vi "Actor Core.vi"(8 "error in":errorcluster, 11 "ThresholdProcess2D in":refnum<class "ThresholdProcessor2D.lvclass">) -> (0 "error out":errorcluster, 3 "Actor out":refnum<class "Actor.lvclass">)   [LabVIEW 2014, in "ThresholdProcessor2D.lvclass"]
doc: "(<B>Filename</B>: Actor Framework.lvlib:Actor.lvclass:Actor Core.vi)\n\nReceives messages to the actor, reacts to them, and initiates any error handling that may shut the actor down.\n\nDescendant classes may override this VI to append parallel tasks for the actor to complete while it handles messages. Overrides use the Call Parent Method node."
uses:
  ThresholdProcessor2D.lvclass
  Framework/Interfaces/Viewable Actor/Viewable Actor.lvclass
  <vilib>/ActorFramework/Actor/Actor.lvclass
  Framework/Interfaces/Observable Actor/Observable Actor.lvclass
  ThresholdProcessor2D Messages/Write Threshold2D Msg/Write Threshold2D Msg.lvclass
  Framework/Processor/AbstractProcessor2D/AbstractProcessor2D.lvclass
  Framework/Model/Data/Data2D/Data2D.lvclass
  Framework/Processor/AbstractProcessor2D/Data2D Cluster.ctl
panel:
  out "Data2D out":dbl[][](graph)
  out "Data2D in":dbl[][](graph)
  out "Stop":bool=TRUE
  in  "Threshold":dbl
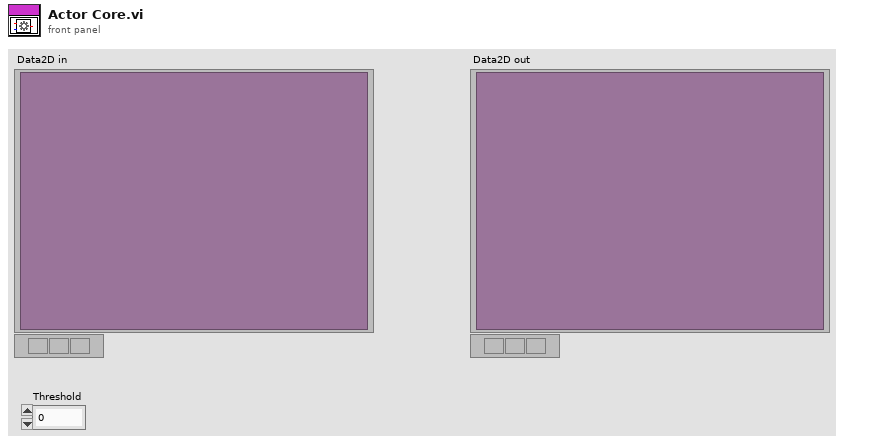
[diagram p1: front panel]
types:
  T1 = typedef "Observable Actor.lvlib/Observable Actor.lvclass/Observer.ctl" = refnum<queue>
  T2 = typedef "AbstractProcessor2D.lvclass/Data2D Cluster.ctl" = cluster{"in":refnum<class "Data2D.lvclass">, "out":refnum<class "Data2D.lvclass">}
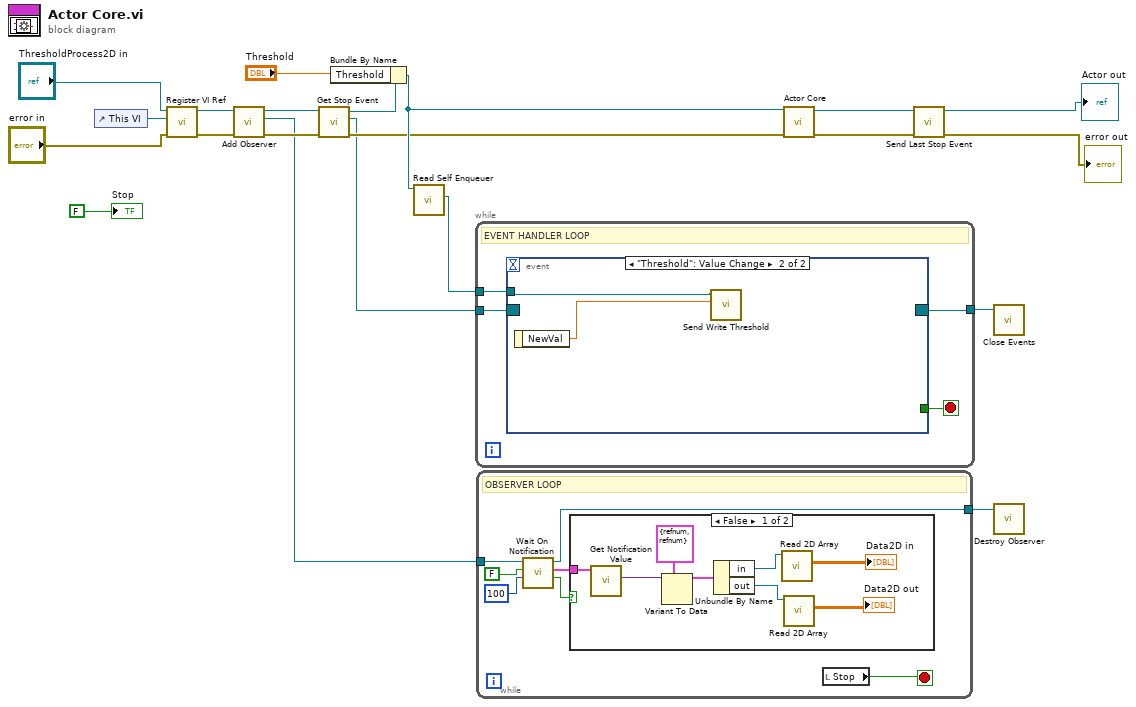
[diagram p0: block diagram]
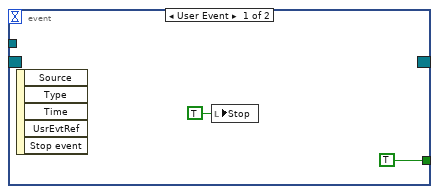
[diagram p3: hidden frame]
diagram:
  n1 = control-ref of="This VI"() -> (w21:refnum<vi>)
  n2 = call "Register VI Ref.vi"("error in (no error)"="error in", "VI ref"=w21, "Viewable Actor in"="ThresholdProcess2D in") -> ("error out"=w5:errorcluster, "Viewable Actor out"=w6:refnum<class "ThresholdProcessor2D.lvclass">)  [unwired: 7 in]
  n3 = call-dynamic "Add Observer.vi"("error in (no error)"=w5, "Observable Actor in"=w6) -> ("error out"=w4:errorcluster, "new observer"=w3:T1, "Observable Actor out"=w7:refnum<class "ThresholdProcessor2D.lvclass">)  [unwired: 7 in]
  n4 = call-dynamic "Get Stop Event.vi"("error in (no error)"=w4, "Observable Actor in"=w7) -> ("error out"=w9:errorcluster, "Events"=w8:refnum<event-registration>, "Observable Actor out"=w10:refnum<class "ThresholdProcessor2D.lvclass">)  [unwired: 7 in]
  n5 = Bundle By Name(cluster=w10, "Threshold"="Threshold") -> (w11:refnum<class "ThresholdProcessor2D.lvclass">)
  n6 = call <vilib>:"Read Self Enqueuer.vi"("Actor"=w11) -> ("Self Enqueuer"=w20:refnum<class "Message Enqueuer.lvclass">)  [unwired: 10 in]
  n7 = while {
    tunnel: w8 -> [w25]
    tunnel: w20 -> [w24]
    tunnel: [w23] -> w2
    stop <- w22 stop-if-true
    # "EVENT HANDLER LOOP"
    n8 = event shown="[1] \"Threshold\": Value Change" {
      selector: w25 -> [_ _]
      dyn-events: [_ _] -> w23
      timeout: _ -> [_ _]
      tunnel: w24 -> [_ w29]
      tunnel: [TRUE _] -> w22
      event User Event {
        n9 = event-data() -> ()  [unwired: 1 in, 5 out]
        n10 = local write "Stop"(TRUE ("Stop")) -> ()
      }
      event "Threshold": Value Change {
        n11 = event-data() -> ("NewVal"=w28:dbl)  [unwired: 1 in]
        n12 = call "Send Write Threshold.vi"("Threshold"=w28, "Message Enqueuer"=w29) -> ()  [unwired: 8 in, 2 out]
      }
    }
  }
  n13 = while {
    tunnel: [w34] -> w1
    tunnel: w3 -> [w35]
    stop <- w36 stop-if-true
    # "OBSERVER LOOP"
    n14 = call "Wait On Notification.vi"("timeout in ms (-1)"=100, "ignore previous (F)"=FALSE, "observer in"=w35) -> ("timed out?"=w30:bool, "notification"=w31:cluster{"value":variant, "name":string}, "observer out"=w34:T1)  [unwired: 5 in, 1 out]
    n15 = case shown="False" w30 {
      tunnel: w31 -> [w44 _]
      frame False {
        n16 = call "Get Notification Value.vi"("notification in"=w44) -> ("data"=w41:variant)  [unwired: 7 in, 1 out]
        n17 = Variant To Data(type=T2 {"in"=refnum, "out"=refnum} ("Cluster"), Variant=w41) -> (data=w39:T2)  [unwired: 1 in, 1 out]
        n18 = Unbundle By Name(w39) -> ("in"=w42:refnum<class "Data2D.lvclass">, "out"=w43:refnum<class "Data2D.lvclass">)
        n19 = call "Read 2D Array.vi"("Data2D in"=w42) -> ("2D Array"=→"Data2D in":dbl[][])  [unwired: 8 in, 2 out]
        n20 = call "Read 2D Array.vi"("Data2D in"=w43) -> ("2D Array"=→"Data2D out":dbl[][])  [unwired: 8 in, 2 out]
      }
      frame True {
      }
    }
    n21 = local read "Stop"() -> (w36:bool)
  }
  n22 = call-parent "Actor Core.vi"("error in"=w9, "Actor in"=w11) -> ("error out"=w13:errorcluster, "Actor out"=w14:refnum<class "Actor.lvclass">)  [unwired: 8 in]
  n23 = call "Send Last Stop Event.vi"("error in (no error)"=w13, "Actor in"=w14) -> ("error out"=→"error out":errorcluster, "Actor  out"=→"Actor out":refnum<class "Actor.lvclass">)  [unwired: 8 in]
  n24 = call "Close Events.vi"("events"=w2) -> ()  [unwired: 11 in]
  n25 = call "Destroy Observer.vi"("observer in"=w1) -> ()  [unwired: 11 in]
  "Stop" <- FALSE ("Stop")
